vi "reset_stage_error (SubVI).vi"(9 "error IO":errorcluster, 10 "reference":refnum<k24>, 11 "deviceKey":string) -> (1 "error IO 2":errorcluster, 2 "new reference":refnum<k24>, 3 "String":string)   [LabVIEW 2016]
uses:
  C:/Users/UsphereLab/Documents/GitHub/Optlev/LabView Code/Examples/Tilt Stage/CmdLib.dll
  Examples/Tilt Stage/CmdLib.dll
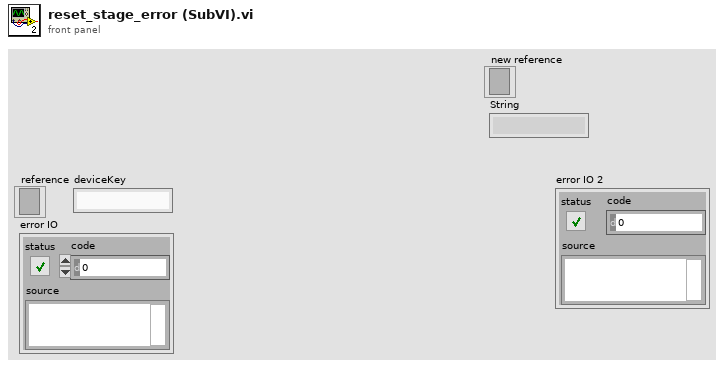
[diagram p1: front panel]
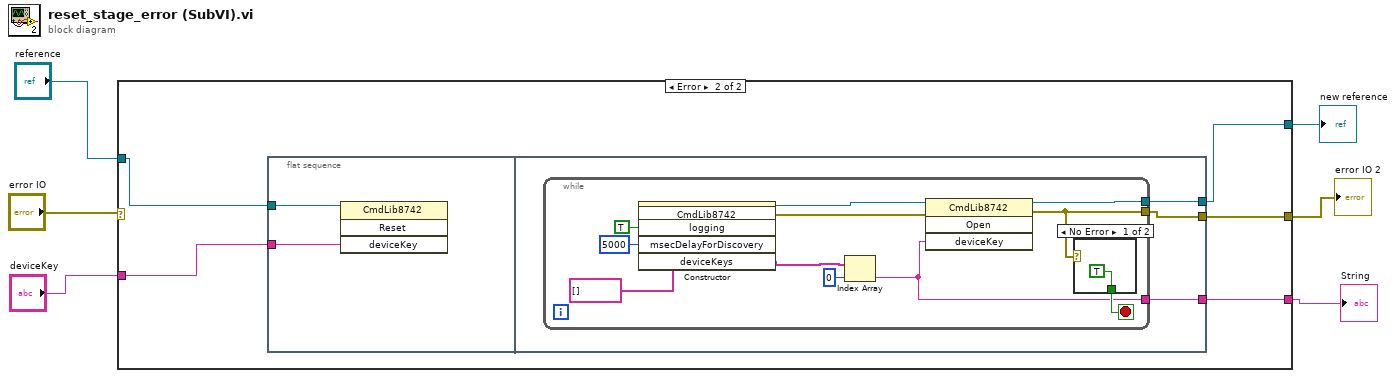
[diagram p0: block diagram]
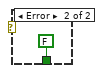
[diagram p3: hidden frame]
diagram:
  n1 = case shown="Error" "error IO" {
    selector: "error IO" -> [w9 _]
    tunnel: "reference" -> [w8 w14]
    tunnel: "deviceKey" -> [w7 w13]
    tunnel: [w9 w12] -> w4
    tunnel: [w8 w11] -> w2
    tunnel: [w7 w10] -> w1
    frame No Error {
    }
    frame Error {
      n2 = flat-sequence {
        tunnel: w14 -> [w16]
        tunnel: w13 -> [w15]
        tunnel: [w19] -> w11
        tunnel: [w18] -> w12
        tunnel: [w17] -> w10
        frame #0 {
          n3 = invoke class="CmdLib8742" method="Reset"(reference=w16, "deviceKey"=w15) -> ()  [unwired: 2 in, 4 out]
        }
        frame #1 {
          n4 = while {
            tunnel: [w26] -> w19
            tunnel: [w24] -> w18
            tunnel: [w20] -> w17
            stop <- w23 stop-if-true
            n5 = constructor class="CmdLib8742"("logging"=TRUE, "msecDelayForDiscovery"=5000, "deviceKeys"=string[] []) -> (reference out=w30:refnum<k24>, error out=w25:errorcluster, "deviceKeys"=w27:string[])  [unwired: 3 in, 3 out]
            n6 = Index Array(array=w27, index=0) -> (element=w20:string)
            n7 = invoke class="CmdLib8742" method="Open"(reference=w30, error in=w25, "deviceKey"=w20) -> (reference out=w26:refnum<k24>, error out=w24:errorcluster)  [unwired: 1 in, 2 out]
            n8 = case shown="No Error" w24 {
              tunnel: [TRUE FALSE] -> w23
              frame No Error {
              }
              frame Error {
              }
            }
          }
        }
      }
    }
  }
  "error IO 2" <- w4
  "new reference" <- w2
  "String" <- w1
